vi "state machine ejemplo.vi"() -> ()   [LabVIEW 2018]
uses:
  States.ctl
panel:
  in  "error in":errorcluster
  out "error out":errorcluster
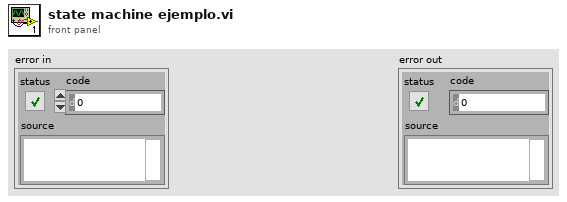
[diagram p1: front panel]
types:
  T1 = typedef "States.ctl" = enum16{"Initialize", "paso 1", "paso 2", "shutdown"}
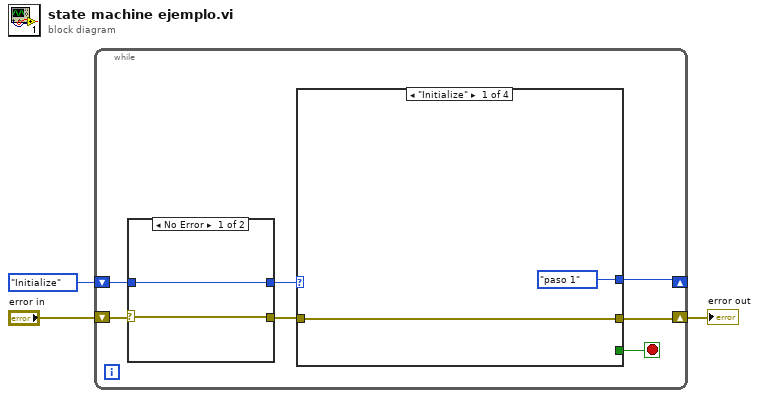
[diagram p0: block diagram]
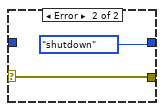
[diagram p2: hidden frame]
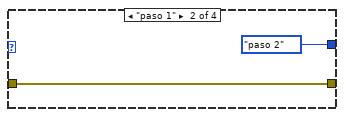
[diagram p3: hidden frame]
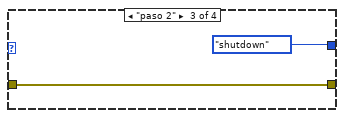
[diagram p4: hidden frame]
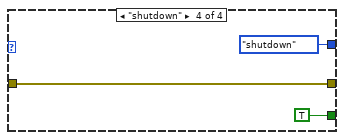
[diagram p5: hidden frame]
diagram:
  n1 = while {
    shift-right: [w6] -> _
    shift-left: States."Initialize" ("States") -> [w8]
    shift-right: [w7] -> w1
    shift-left: "error in" -> [w4]
    stop <- w5 stop-if-true
    n2 = case shown="No Error" w4 {
      selector: w4 -> [w11 w13]
      tunnel: w8 -> [w12 _]
      tunnel: [w12 States."shutdown" ("States")] -> w10
      tunnel: [w11 w13] -> w9
      frame No Error {
      }
      frame Error {
      }
    }
    n3 = case shown="\"Initialize\"" w10 {
      tunnel: w9 -> [w16 w17 w19 w22]
      tunnel: [w16 w17 w19 w22] -> w7
      tunnel: [States."paso 1" ("States") States."paso 2" ("States") States."shutdown" ("States") States."shutdown" ("States")] -> w6
      tunnel: [_ _ _ TRUE] -> w5
      frame "Initialize" {
      }
      frame "paso 1" {
      }
      frame "paso 2" {
      }
      frame "shutdown" {
      }
    }
  }
  "error out" <- w1
